vi "Example_instrument_detection_usecase.vi"() -> ()   [LabVIEW 2020]
panel:
  out "2400 Address string":string
  in  "2400 Address":u32
  out "2400 detected":bool
  out "error IO":errorcluster
  out "Sampled Output":string
  out "3457A Address string":string
  out "4275A Address string":string
  in  "error in (no error)":errorcluster
  out "3457A detected":bool
  out "4275A detected":bool
  in  "4275A Address":u32
  in  "3457A Address":u32
  out "Sampled Output":string
  out "Sampled Output":string
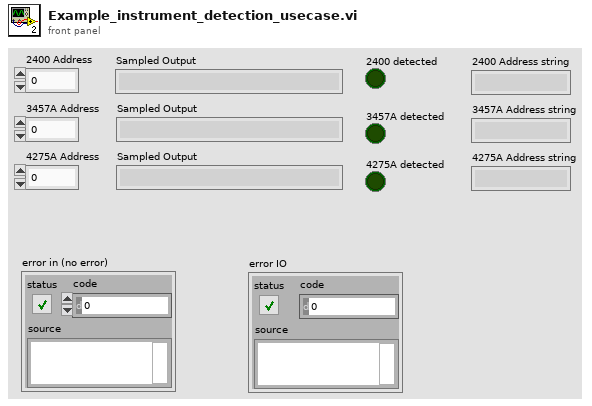
[diagram p1: front panel]
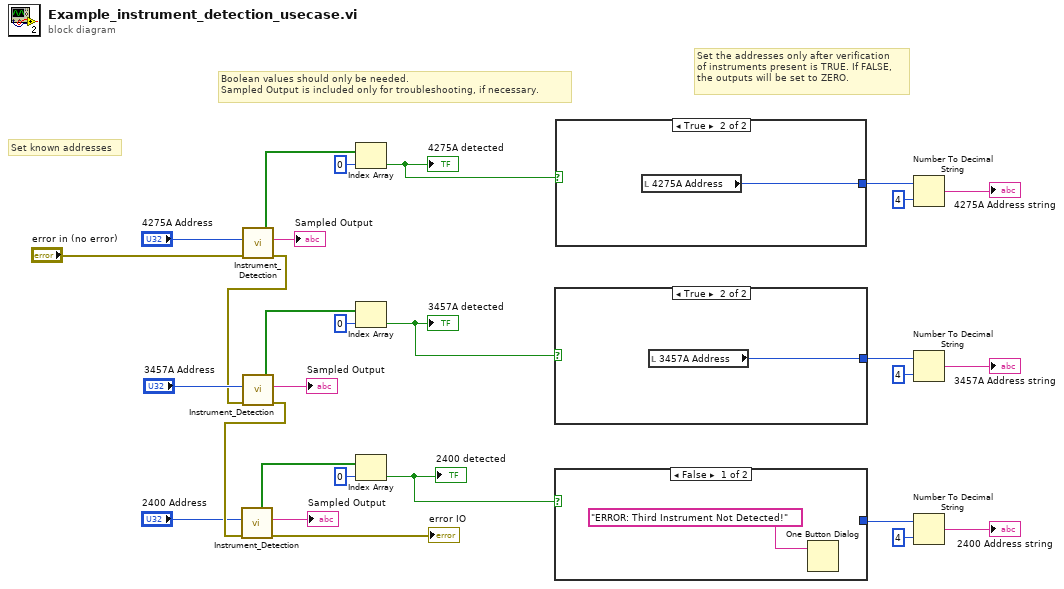
[diagram p0: block diagram]
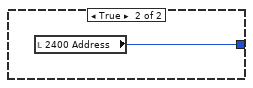
[diagram p2: hidden frame]
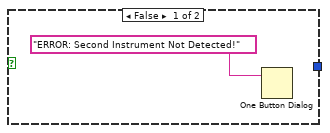
[diagram p3: hidden frame]
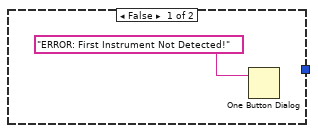
[diagram p4: hidden frame]
diagram:
  # "Set the addresses only after verification \nof instruments present is TRUE. If FALSE,\nthe outputs will be set to ZERO."
  # "Boolean values should only be needed.\nSampled Output is included only for troubleshooting, if necessary."
  # "Set known addresses"
  n1 = call "Instrument_Detection.vi"("error in (no error)"="error in (no error)", "GPIB Address"="4275A Address") -> ("error IO"=w19:errorcluster, "ID"=→"Sampled Output":string, "Instrument detected?"=w24:bool[])  [unwired: 7 in]
  n2 = call "Instrument_Detection.vi"("error in (no error)"=w19, "GPIB Address"="3457A Address") -> ("error IO"=w10:errorcluster, "ID"=→"Sampled Output":string, "Instrument detected?"=w22:bool[])  [unwired: 7 in]
  n3 = call "Instrument_Detection.vi"("error in (no error)"=w10, "GPIB Address"="2400 Address") -> ("error IO"=→"error IO":errorcluster, "ID"=→"Sampled Output":string, "Instrument detected?"=w8:bool[])  [unwired: 7 in]
  n4 = Index Array(array=w24, index=0) -> (element=w18:bool)
  "4275A detected" <- w18
  n5 = Index Array(array=w22, index=0) -> (element=w17:bool)
  "3457A detected" <- w17
  n6 = Index Array(array=w8, index=0) -> (element=w2:bool)
  "2400 detected" <- w2
  n7 = case shown="True" w17 {
    tunnel: [_ w30] -> w13
    frame False {
      n8 = One Button Dialog(message="ERROR: Second Instrument Not Detected!") -> ()  [unwired: 1 in, 1 out]
    }
    frame True {
      n9 = local read "3457A Address"() -> (w30:u32)
    }
  }
  n10 = case shown="False" w2 {
    tunnel: [_ w32] -> w5
    frame False {
      n11 = One Button Dialog(message="ERROR: Third Instrument Not Detected!") -> ()  [unwired: 1 in, 1 out]
    }
    frame True {
      n12 = local read "2400 Address"() -> (w32:u32)
    }
  }
  n13 = case shown="True" w18 {
    tunnel: [_ w34] -> w16
    frame False {
      n14 = One Button Dialog(message="ERROR: First Instrument Not Detected!") -> ()  [unwired: 1 in, 1 out]
    }
    frame True {
      n15 = local read "4275A Address"() -> (w34:u32)
    }
  }
  n16 = Number To Decimal String(number=w16, width (-)=i16 4) -> (decimal integer string=→"4275A Address string":string)
  n17 = Number To Decimal String(number=w13, width (-)=i16 4) -> (decimal integer string=→"3457A Address string":string)
  n18 = Number To Decimal String(number=w5, width (-)=i16 4) -> (decimal integer string=→"2400 Address string":string)
